vi "add_meas_date.vi"(0 "Data":timestamp, 1 "measurment to add":T1, 2 "to date?":bool, 3 "new?":bool) -> ()   [LabVIEW 2012]
uses:
  meas_date.vi
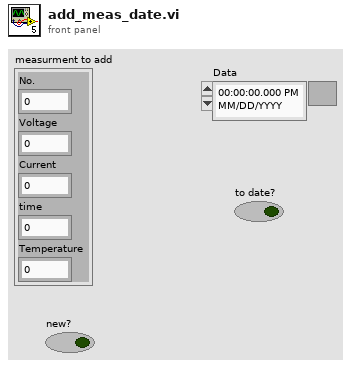
[diagram p1: front panel]
types:
  T1 = cluster{"No.":u64, "Voltage":dbl, "Current":dbl, "time":dbl, "Temperature":dbl}
  T2 = cluster{"VCT measurment's date":cluster{"No.":u64, "Voltage":dbl, "Current":dbl, "time":dbl, "Temperature":dbl}[], "Data":timestamp}[]
  T3 = cluster{"VCT measurment's date":cluster{"No.":u64, "Voltage":dbl, "Current":dbl, "time":dbl, "Temperature":dbl}[], "Data":timestamp}
  T4 = cluster{"No.":u64, "Voltage":dbl, "Current":dbl, "time":dbl, "Temperature":dbl}[]
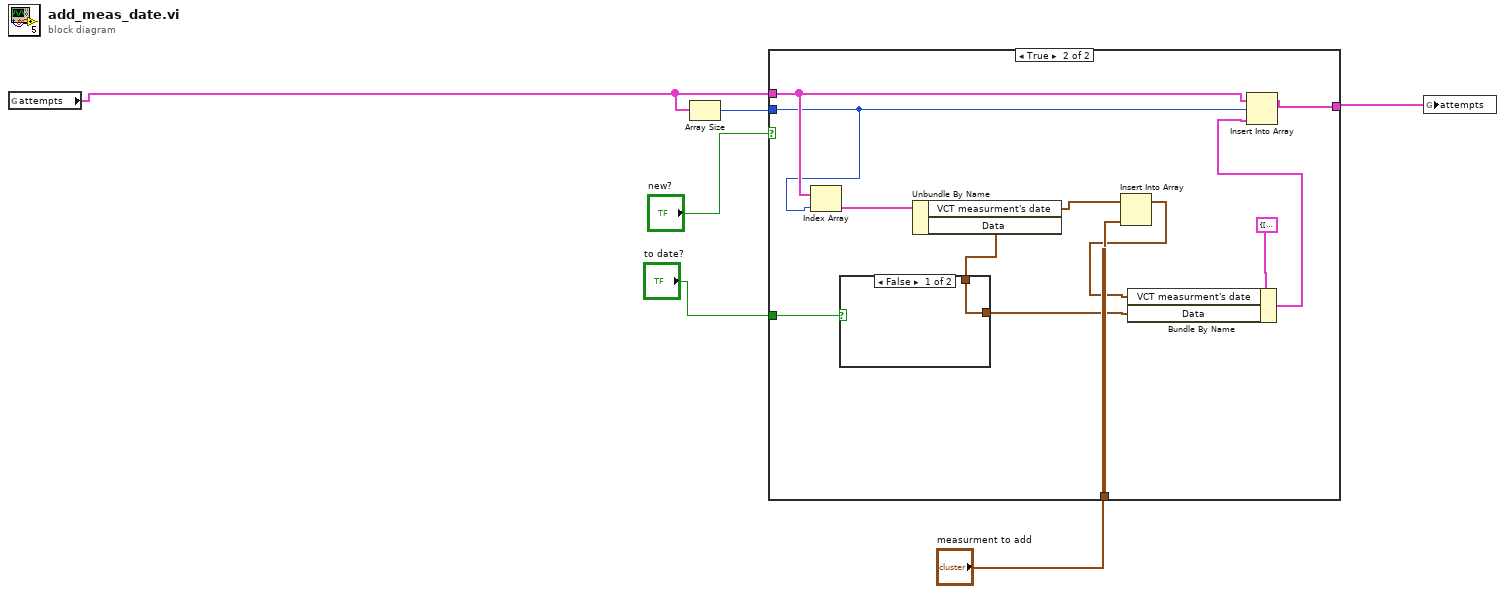
[diagram p0: block diagram]
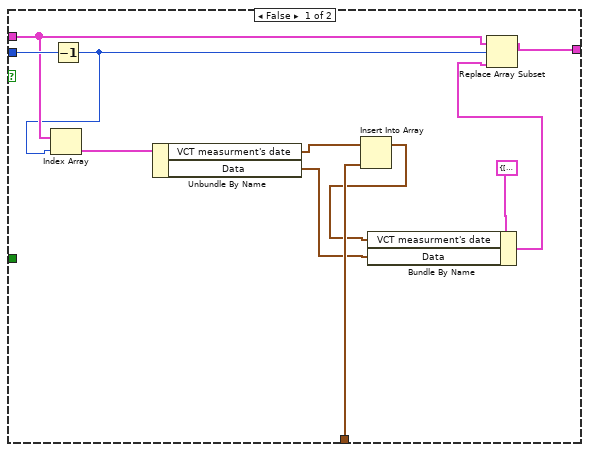
[diagram p2: hidden frame]
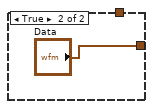
[diagram p3: hidden frame]
diagram:
  n1 = global read "meas_date.vi" "attempts"() -> (w2:T2)
  n2 = Array Size(array=w2) -> (size(s)=w4:i32)
  n3 = case shown="True" "new?" {
    tunnel: [w17 w29] -> w6
    tunnel: w2 -> [w14 w27]
    tunnel: w4 -> [w16 w21]
    tunnel: "measurment to add" -> [w11 w25]
    tunnel: "to date?" -> [_ w20]
    frame False {
      n4 = Decrement(x=w16) -> (x-1=w13:i32)
      n5 = Index Array(array=w14, index=w13) -> (element=w15:T3)
      n6 = Unbundle By Name(w15) -> ("VCT measurment's date"=w12:T4, "Data"=w9:timestamp)
      n7 = Insert Into Array(array=w12, new element=w11) -> (w8:T4)  [unwired: 1 in]
      n8 = Bundle By Name(cluster=T3 {"VCT measurment's date"=[], "Data"=timestamp(0 s since 1904-01-01)} ("test"), "VCT measurment's date"=w8, "Data"=w9) -> (w7:T3)
      n9 = Replace Array Subset(array=w14, new element=w7, index=w13) -> (w17:T2)
    }
    frame True {
      n10 = Index Array(array=w27, index=w21) -> (element=w28:T3)
      n11 = Unbundle By Name(w28) -> ("VCT measurment's date"=w26:T4, "Data"=w18:timestamp)
      n12 = case shown="False" w20 {
        tunnel: [w30 "Data"] -> w19
        tunnel: w18 -> [w30 _]
        frame False {
        }
        frame True {
        }
      }
      n13 = Insert Into Array(array=w26, new element=w25) -> (w23:T4)  [unwired: 1 in]
      n14 = Bundle By Name(cluster=T3 {"VCT measurment's date"=[], "Data"=timestamp(0 s since 1904-01-01)} ("test"), "VCT measurment's date"=w23, "Data"=w19) -> (w22:T3)
      n15 = Insert Into Array(array=w27, index=w21, new element=w22) -> (w29:T2)
    }
  }
  n16 = global write "meas_date.vi" "attempts"(w6) -> ()
